vi "get VTK x Offset.vi"(8 "error in (no error)":errorcluster) -> (0 "error out":errorcluster, 3 "function return":dbl)   [LabVIEW 2019, in "libConvectionDiffusionWrapper.lvlib"]
doc: "double getVTK_xOffset();"
uses:
  libConvectionDiffusionWrapper.lvlib
  libConvectionDiffusionWrapper.so
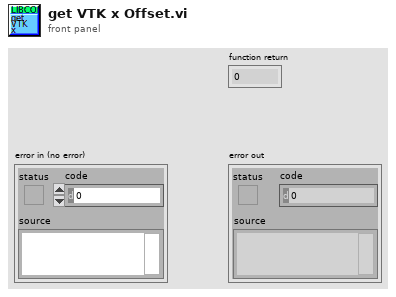
[diagram p1: front panel]
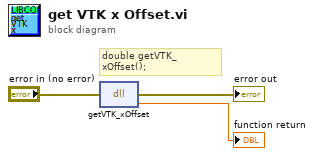
[diagram p0: block diagram]
diagram:
  # "double getVTK_xOffset();"
  n1 = dll-call lib="home/paul/Schreibtisch/Convection_diffusion/LabView/lib/libConvectionDiffusionWrapper.*" fn="getVTK_xOffset"(error in="error in (no error)") -> (error out=→"error out":errorcluster, →"function return":dbl)  [unwired: 2 in, 1 out]
